vi "CountTilesInArray.vi"(9 "Tile":u16(ring), 10 "Hand":u16[](array[ring])) -> (2 "Count":u16)   [LabVIEW 2025]
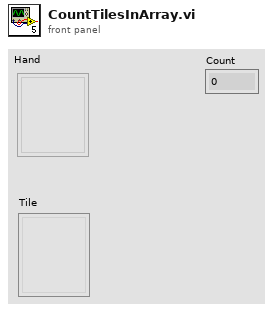
[diagram p1: front panel]
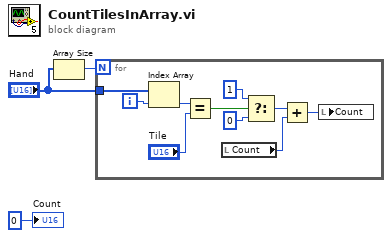
[diagram p0: block diagram]
diagram:
  n1 = Array Size(array="Hand") -> (size(s)=w3:i32)
  n2 = for {
    N: w3 -> [_]
    tunnel: "Hand" -> [w13]
    i -> [w12]
    n3 = Index Array(array=w13, index=w12) -> (element=w10:u16)
    n4 = Equal?(x=w10, y="Tile") -> (x = y?=w11:bool)
    n5 = local read "Count"() -> (w4:u16)
    n6 = Select(t=1, s=w11, f=0) -> (s? t:f=w8:i32)
    n7 = Add(x=w8, y=w4) -> (x+y=w5:i32)
    n8 = local write "Count"(w5) -> ()
  }
  "Count" <- 0
